vi "Talker.vi"(0 "Arithmetic_Operations in":refnum<class "Arithmetic_Operations.lvclass">, 5 "Subpanel Ref":refnum<vi>, 11 "Error In":errorcluster) -> (4 "Arithmetic_Operations out":refnum<class "Arithmetic_Operations.lvclass">, 15 "Error Out":errorcluster)   [LabVIEW 2020, in "Arithmetic_Operations.lvclass"]
uses:
  Arithmetic_Operations.lvclass
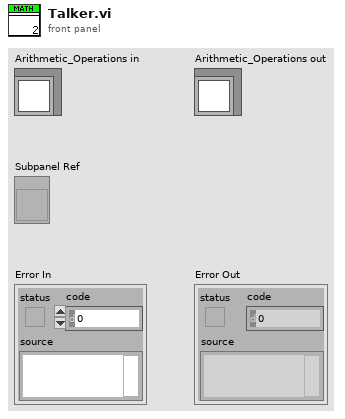
[diagram p1: front panel]
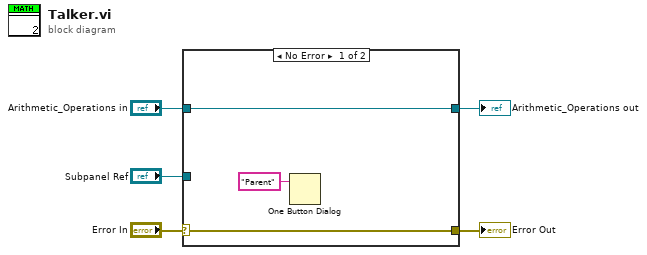
[diagram p0: block diagram]
diagram:
  n1 = case shown="No Error" "Error In" {
    selector: "Error In" -> [w7 w10]
    tunnel: [w7 w10] -> w4
    tunnel: [w8 w9] -> w2
    tunnel: "Arithmetic_Operations in" -> [w8 w9]
    tunnel: "Subpanel Ref" -> [_ _]
    frame No Error {
      n2 = One Button Dialog(message="Parent") -> ()  [unwired: 1 in, 1 out]
    }
    frame Error {
    }
  }
  "Error Out" <- w4
  "Arithmetic_Operations out" <- w2
